vi "Shared Variable Client - Front Panel Binding.vi"() -> ()   [LabVIEW 2016]
doc: "This client VI connects to Shared Variable Server.vi by binding its front panel charts to the shared variables hosted by the server."
panel:
  out "Monitor Value 2":dbl(graph)
  out "Monitor Value 1":dbl(graph)
  in  "Stop":bool
  # "Overview: Demonstrates the use of Front Panel Binding to read shared variable data from a server VI.\nRequirements: Windows\nInstructions:\n1. Make sure Shared Variable Server.vi is already running.\n2. Run this VI. It will read the values of the sever shared variables through bindings configured on the charts themselves.\n3. Click Stop to stop the VI."
  # "Note: To configure front panel shared variable binding, right click a control or indicator and select Properties. On the Data Binding page in the Properties dialog, select Shared Variable Engine (NI-PSP). Then, browse to the appropriate variable Path. If you selected a valid variable, the triangular PSP LED attached to the upper-right corner of the control or indicator will turn green when the VI runs.\n\nIf you ever change the name of the server variable (or the name of its owning library), you will need to manually change this front panel binding as well."
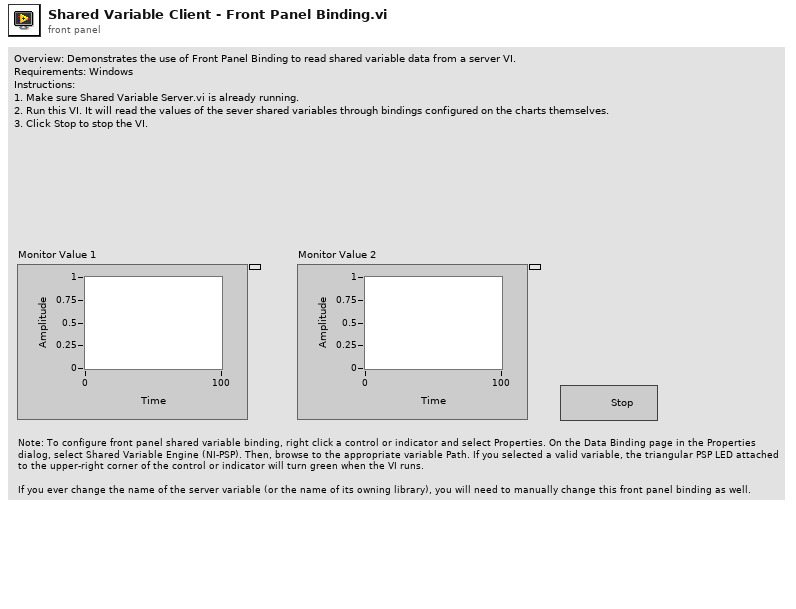
[diagram p1: front panel]
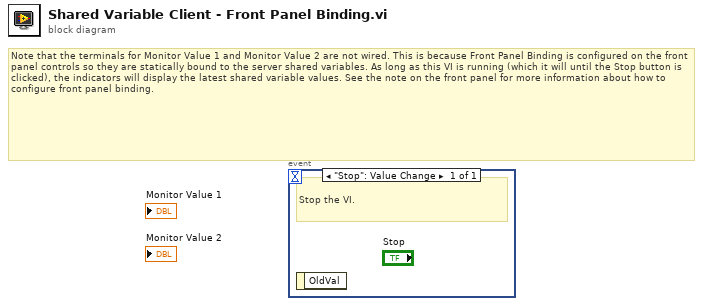
[diagram p0: block diagram]
diagram:
  # "Note that the terminals for Monitor Value 1 and Monitor Value 2 are not wired. This is because Front Panel Binding is configured on the front panel controls so they are statically bound to the server shared variables. As long as this VI is running (which it will until the Stop button is clicked), the indicators will display the latest shared variable values. See the note on the front panel for more information about how to configure front panel binding."
  n1 = event shown="[0] \"Stop\": Value Change" {
    selector: _ -> [_]
    dyn-events: _ -> [_]
    timeout: _ -> [_]
    event "Stop": Value Change {
      # "Stop the VI."
      n2 = event-data() -> ()  [unwired: 1 in, 1 out]
    }
  }
